vi "Lidar Camera System V2.vi"() -> ()   [LabVIEW 2017]
doc: "This example project provides a library of VIs that work together to wrap various ethernet packet sniffing functions available from WinPcap, a Windows packet capture program.\n\nNote: You must install WinPcap before running this example. You can download WinPcap from www.winpcap.org.\n\nThis VI reads ethernet packets. It outputs the raw data for the packet as a hexadecimal string. It also parses out the ethernet and IP header information, as well as timestamp information for each packet.\n\nThis VI also enumerates all the ethernet adapters on your system and allows you interactively to select between the various adapters.\n\nPlease note that this project is for demonstration purposes only. It was designed to demonstrate one method in which LabVIEW can be used to interface with external software utilities (such as WinPcap). NI Engineers can only address questions on how to call external code from LabVIEW, not the contents of each call demonstrated in this example. In addition, we cannot guarantee that the software will work with newer versions of the external software package."
uses:
  lvwpcap.lvlib
panel:
  out "Filtered Co-ordinates":T1(array[cluster])
  out "3D LIDAR Data":refnum<vi>(3d-picture)
  out "Colour Map":dbl[][](graph)
  in  "No. Points Plotted":i32
  in  "Tab Control":T2(tab)
  in  "Adapters":i32(listbox)
  out "raw data":string
  out "timestamp":cluster{"tv_sec":u32, "tv_usec":u32}
  out "packets":i32
  out "Packet Length":i32
  out "Stored Packet":string
  out "Discarded Packet":string
  out "Identifier":string
  out "Data Points":T3(array[cluster])
  out "Filtered Data (First Filter)":T4(array[cluster])
  out "Coordinates":T1(array[cluster])
  out "Stored Data":T1(array[cluster])
  out "size":i32
  out "Reached Size":bool
  in  "stop":bool
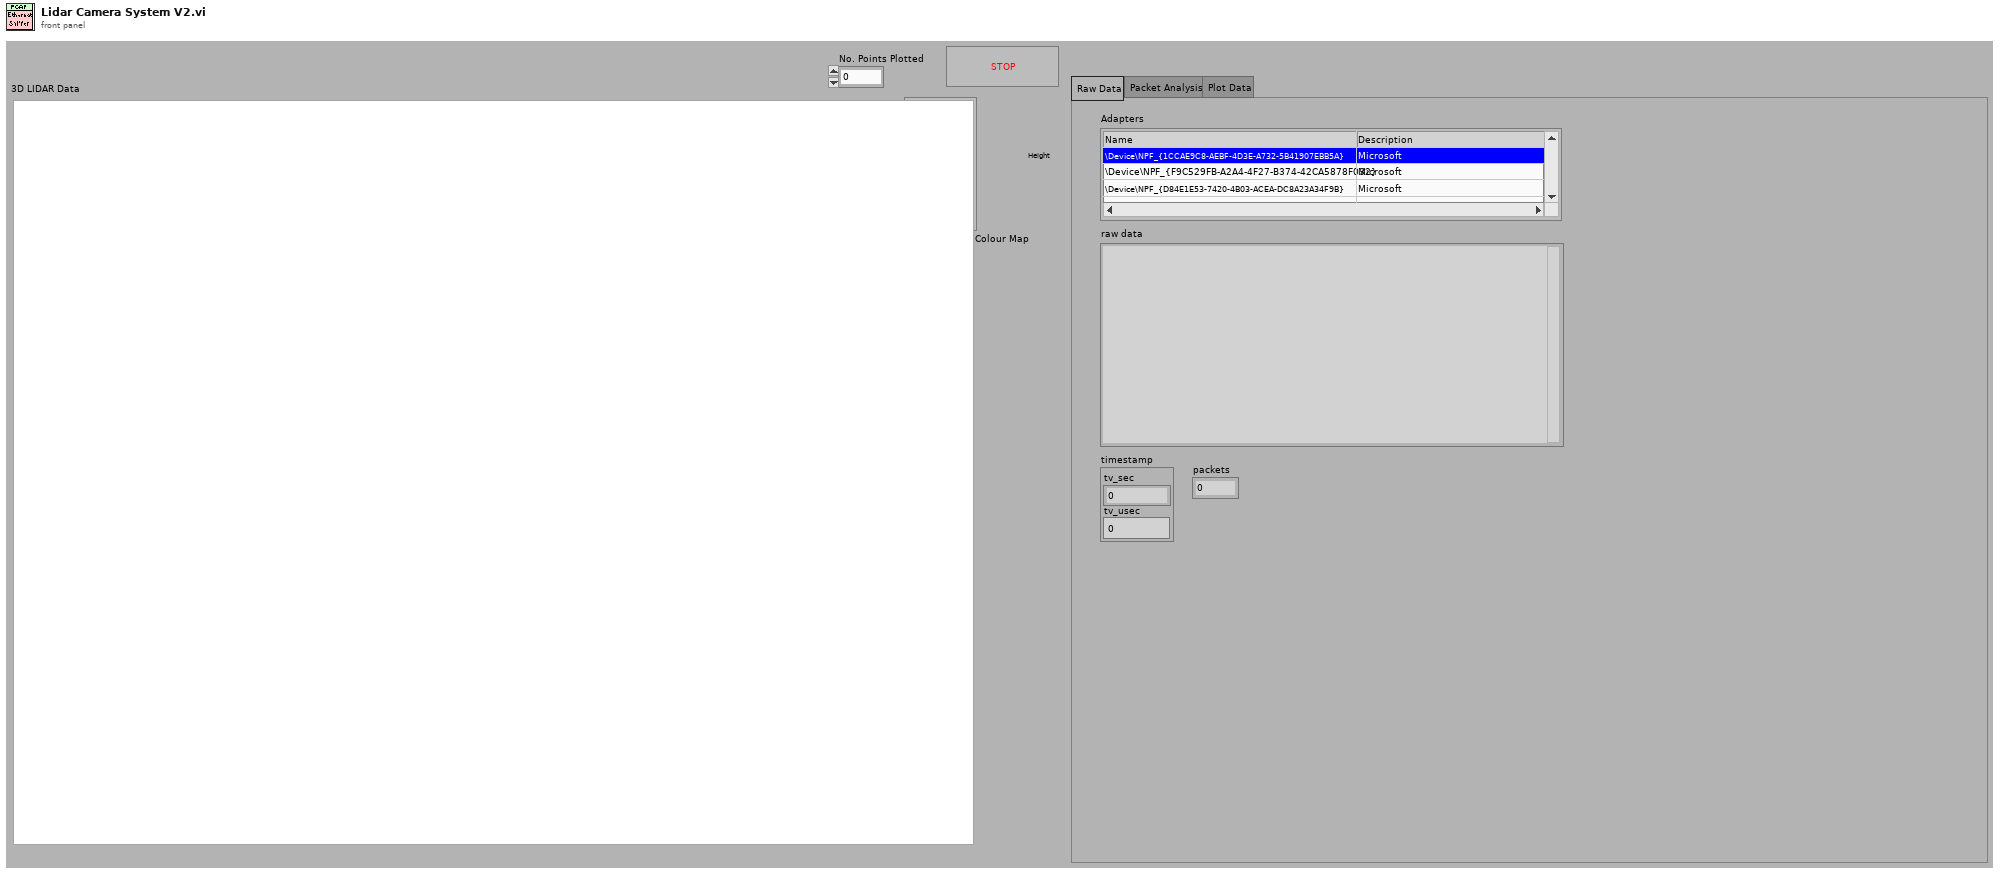
[diagram p1: front panel]
types:
  T1 = cluster{"X":dbl, "Y":dbl, "Z":dbl, "Reflectivity":dbl}[]
  T2 = enum32{"Raw Data", "Packet Analysis", "Plot Data"}
  T3 = cluster{"Azimuth Angle":dbl, "Distance":dbl, "Reflectivity":dbl}[]
  T4 = cluster{"Verticle Angle":dbl, "Azimuth Angle":dbl, "Distance":dbl, "Reflectivity":dbl}[]
  T5 = enum16{"Store Data", "Check Data Size", "Plot Data", "Reinitialise"}
  T6 = enum16{"Check Data", "Check Identifier", "Extract Data", "Filter Data", "Convert to Co-ordinates", "Filter Co-ordinates"}
  T7 = enum16{"Overall", "Per Primitive", "Per Vertex", "Binding Off"}
  T8 = typedef "LVRGBAColorTypeDef.ctl" = cluster{"Red":sgl, "Green":sgl, "Blue":sgl, "Alpha":sgl}
  T9 = enum16{"Check Data", "Check Identifier", "Convert to Hex", "Convert to XYZ", "Check Coords"}
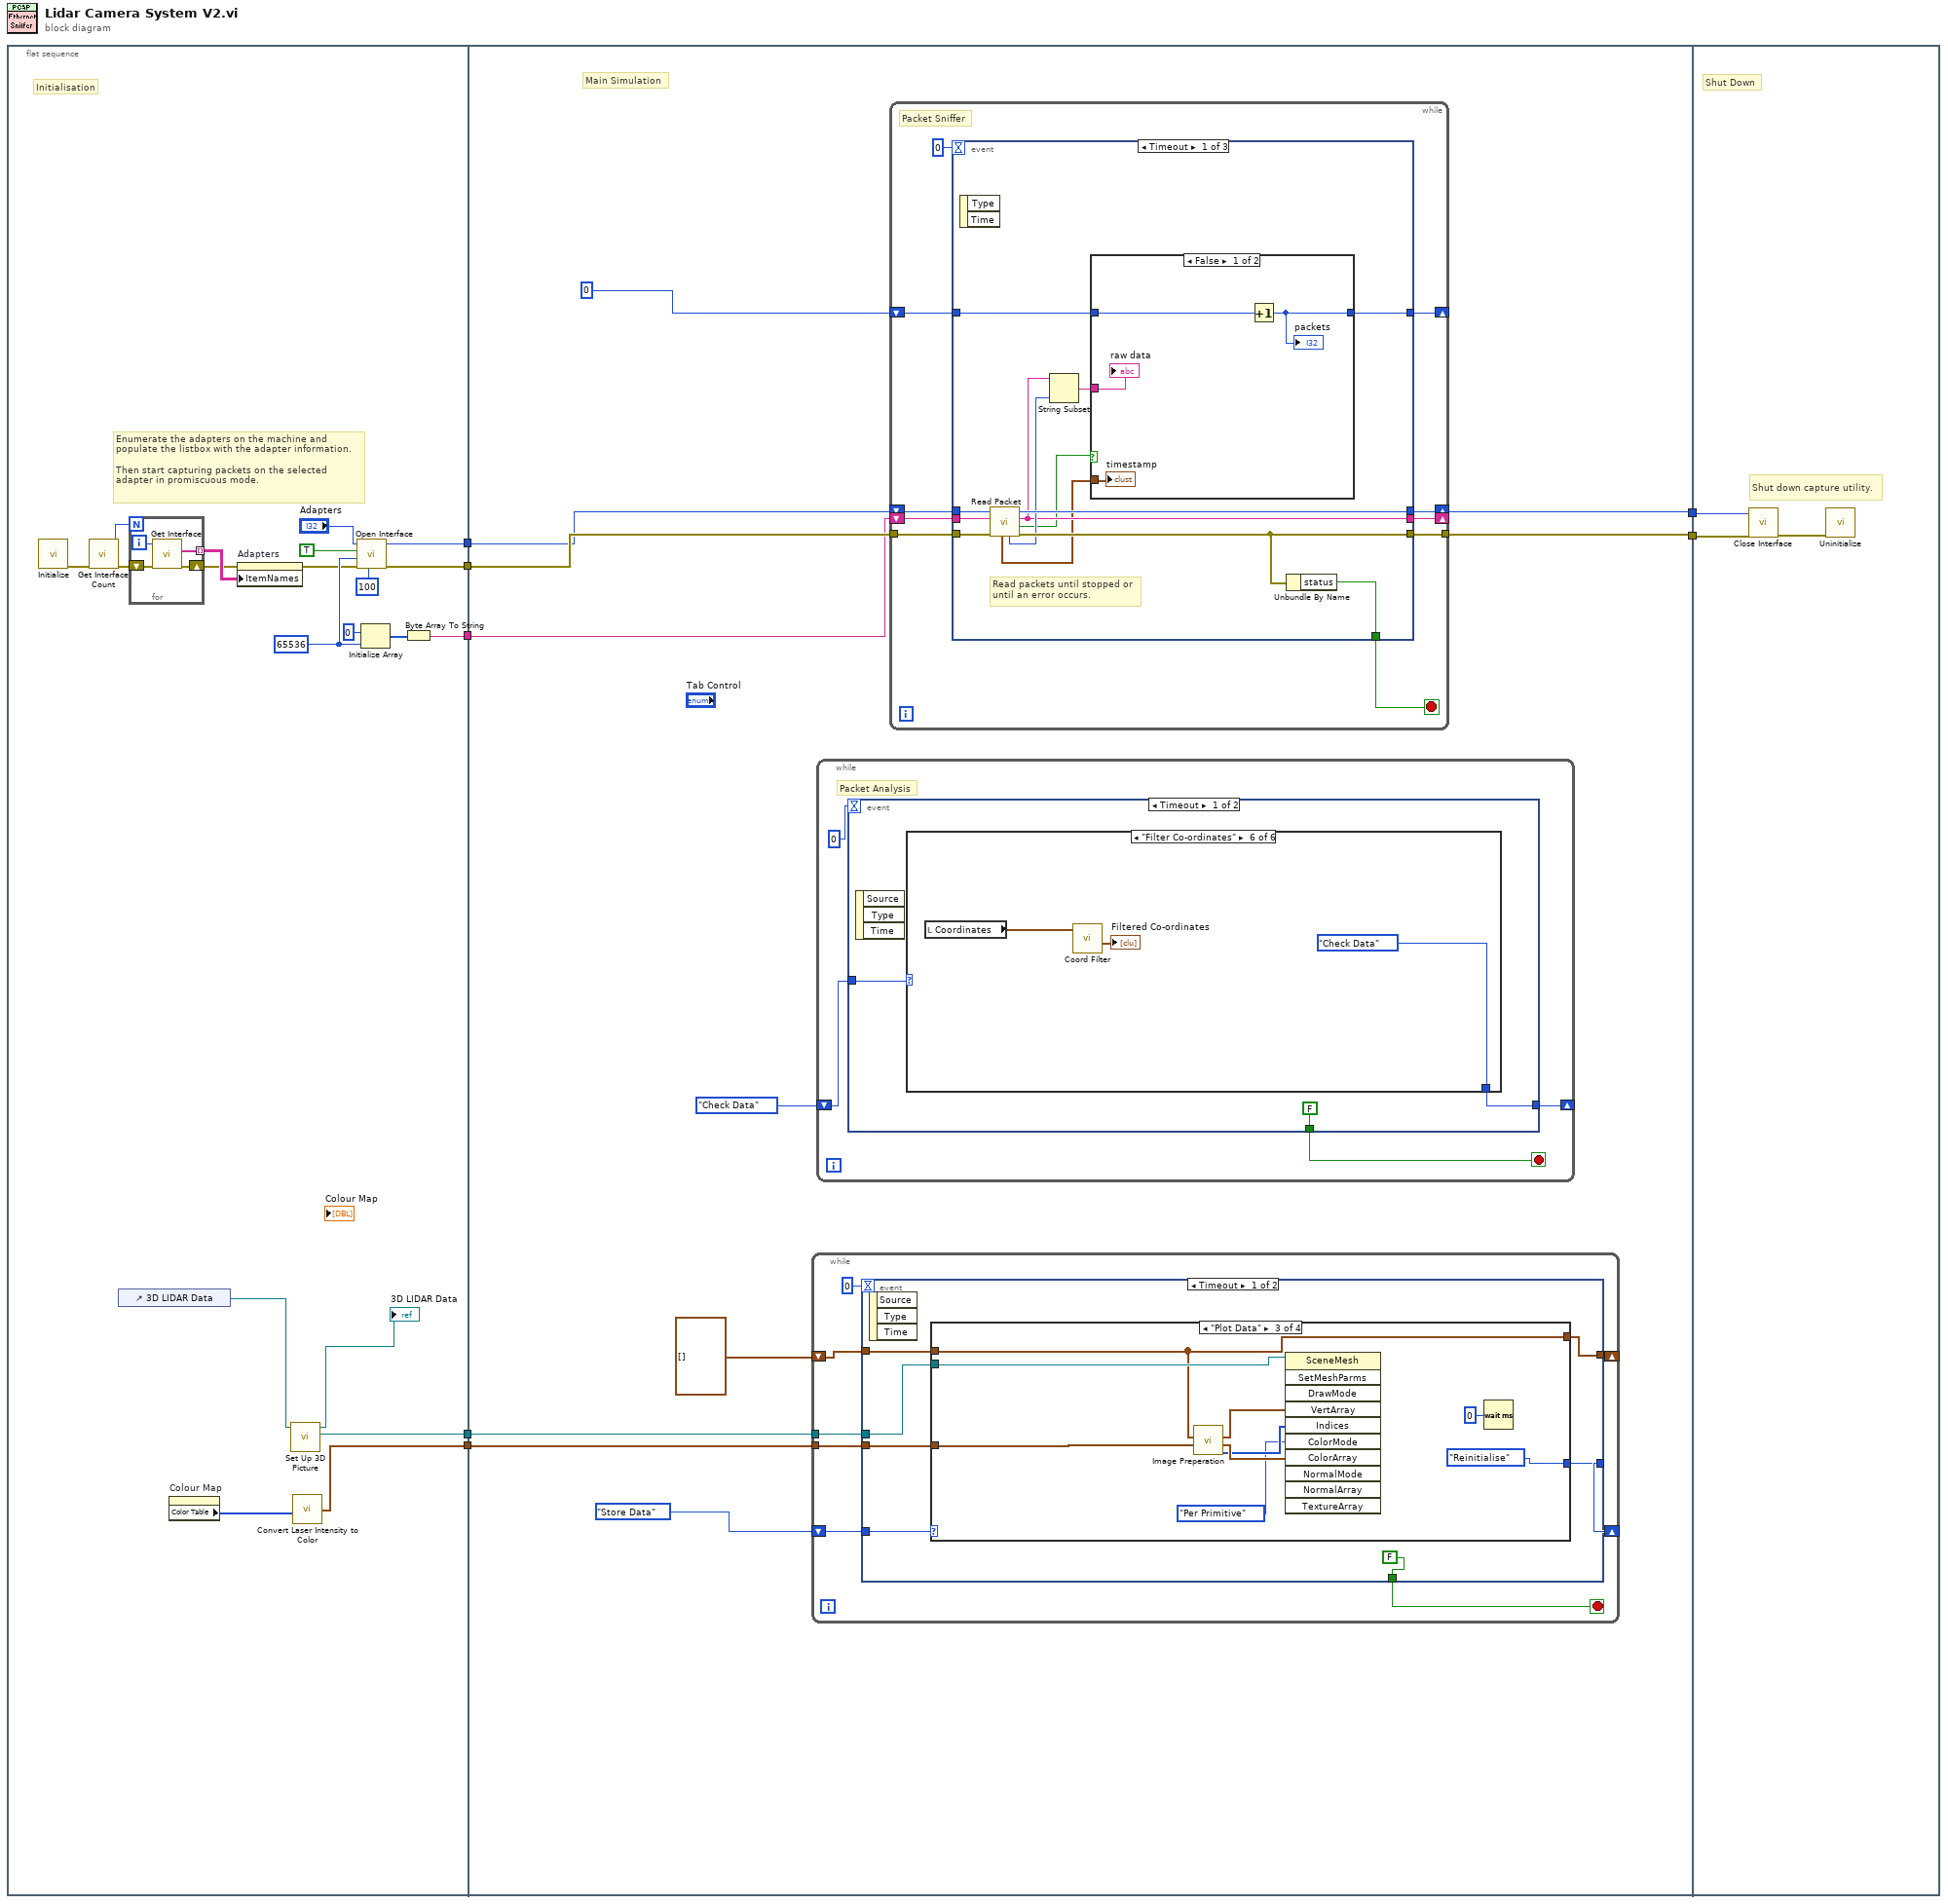
[diagram p0: block diagram]
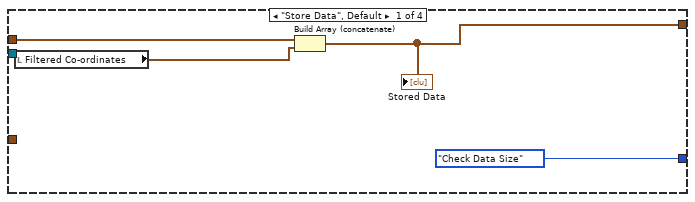
[diagram p2: hidden frame]
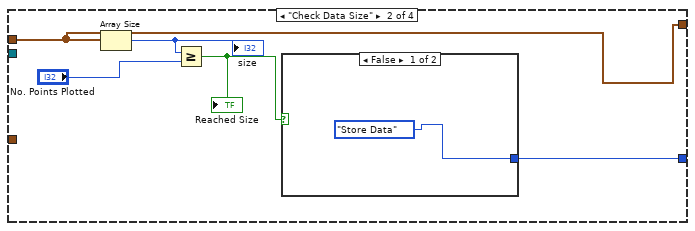
[diagram p3: hidden frame]
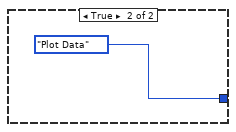
[diagram p4: hidden frame]
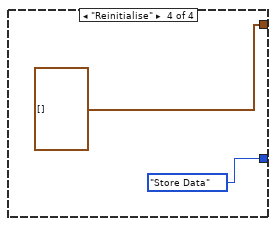
[diagram p5: hidden frame]
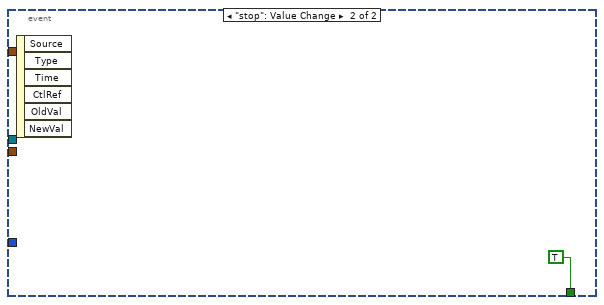
[diagram p6: hidden frame]
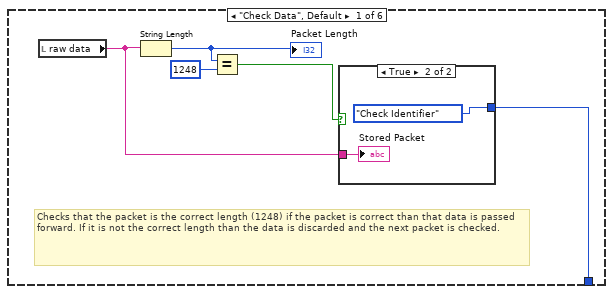
[diagram p7: hidden frame]
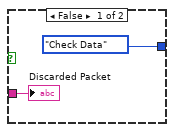
[diagram p8: hidden frame]
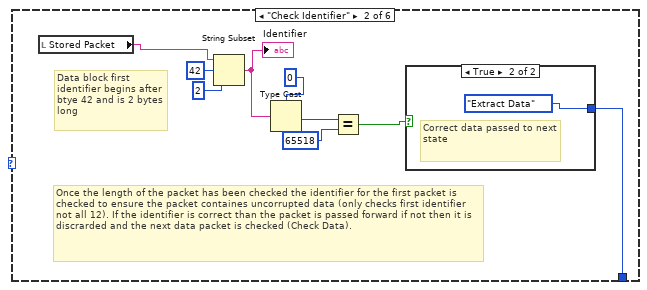
[diagram p9: hidden frame]
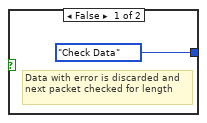
[diagram p10: hidden frame]
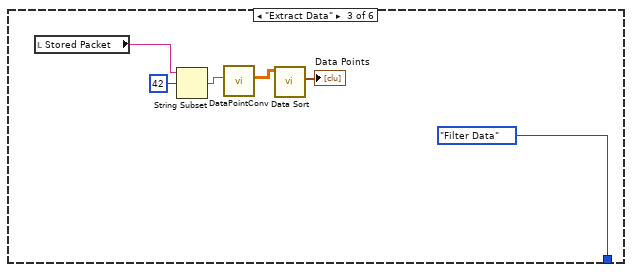
[diagram p11: hidden frame]
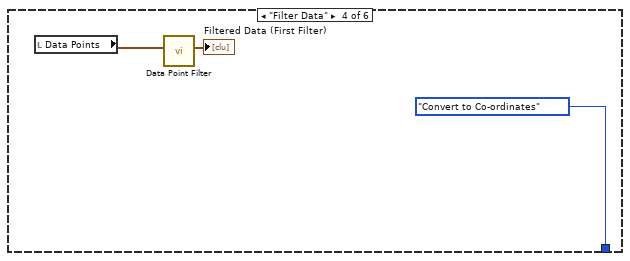
[diagram p12: hidden frame]
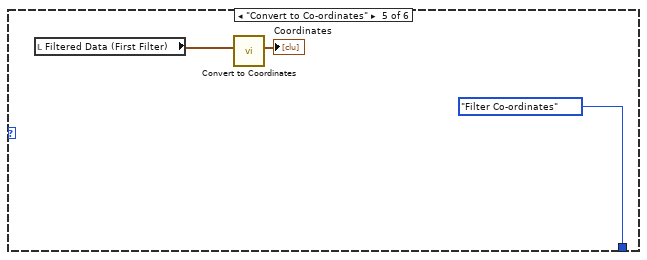
[diagram p13: hidden frame]
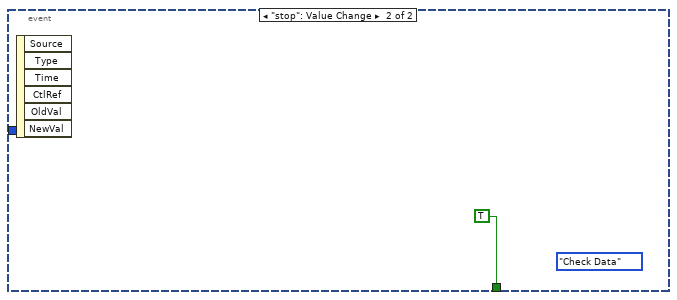
[diagram p14: hidden frame]
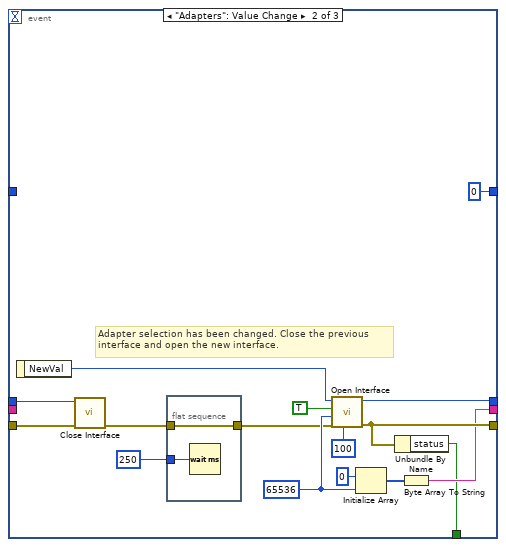
[diagram p16: hidden frame]
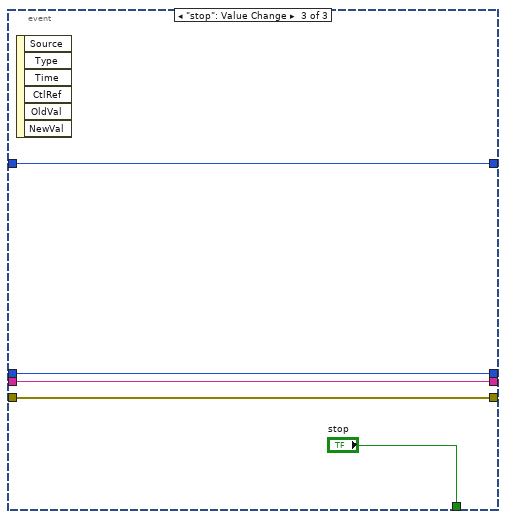
[diagram p17: hidden frame]
diagram:
  n1 = flat-sequence {
    tunnel: [w27] -> w7
    tunnel: [w26] -> w6
    tunnel: [w22] -> w5
    tunnel: [w11] -> w2
    tunnel: [w10] -> w1
    tunnel: w7 -> [w41]
    tunnel: w6 -> [w42]
    tunnel: w5 -> [w40]
    tunnel: [w39] -> w4
    tunnel: [w38] -> w3
    tunnel: w2 -> [w33]
    tunnel: w1 -> [w32]
    tunnel: w4 -> [w177]
    tunnel: w3 -> [w176]
    frame #0 {
      w25 = 65536 ("capture_size (65536)")
      # "Initialisation"
      # "Enumerate the adapters on the machine and\npopulate the listbox with the adapter information.\n\nThen start capturing packets on the selected\nadapter in promiscuous mode."
      n2 = call "Initialize.vi"() -> ("error out"=w20:errorcluster)  [unwired: 11 in]
      n3 = call "Get Interface Count.vi"("error in (no error)"=w20) -> ("error out"=w19:errorcluster, "count"=w18:i32)  [unwired: 9 in]
      n4 = control-ref of="3D LIDAR Data"() -> (w9:refnum<vi>)
      n5 = for {
        N: w18 -> [_]
        shift-right: [w30] -> w14
        shift-left: w19 -> [w31]
        tunnel: [w28] -> w16 mode=indexing
        i -> [w29]
        n6 = call "Get Interface.vi"("error in (no error)"=w31, "index"=w29) -> ("error out"=w30:errorcluster, "lvwpcap_interface_array"=w28:string[])  [unwired: 8 in]
      }
      n7 = property on="Colour Map" class="IntGraph (strict)"() -> ("Color Table"=w12:u32[])  [unwired: 2 in, 2 out]
      n8 = property on="Adapters" class="MCListbox (strict)"(error in=w14, "ItemNames"=w16) -> (error out=w13:errorcluster)  [unwired: 1 in, 1 out]
      n9 = call <instrlib>:"Set Up 3D Picture.vi"("3D Picture Control In"=w9) -> ("Mesh Out"=w11:refnum<vi>, "Scene Out"=→"3D LIDAR Data":refnum<vi>)  [unwired: 9 in]
      n10 = call <instrlib>:"Convert Laser Intensity to Color.vi"("Color Table"=w12) -> ("Color Array"=w10:T8[])  [unwired: 8 in]
      n11 = call "Open Interface.vi"("read_timeout (1000)"=100, "error in (no error)"=w13, "capture_size (65536)"=w25, "promiscuous mode (T)"=TRUE, "adapter (0)"="Adapters") -> ("error out"=w26:errorcluster, "pcap reference"=w27:u32)  [unwired: 5 in]
      n12 = Initialize Array(u8 0, w25) -> (w23:u8[])
      n13 = Byte Array To String(unsigned byte array=w23) -> (string=w22:string)
    }
    frame #1 {
      # "Main Simulation"
      n14 = while {
        shift-right: [w45] -> _
        shift-left: T5."Store Data" -> [w48]
        shift-right: [w46] -> _
        shift-left: cluster{dbl, dbl, dbl, dbl}[] [] -> [w47]
        tunnel: w33 -> [w44]
        tunnel: w32 -> [w43]
        stop <- w49 stop-if-true
        n15 = event shown="[0] Timeout" {
          selector: _ -> [_ _]
          dyn-events: _ -> [_ _]
          timeout: 0 -> [_ _]
          tunnel: [FALSE TRUE] -> w49
          tunnel: w48 -> [w56 _]
          tunnel: w47 -> [w55 _]
          tunnel: [w54 _] -> w46
          tunnel: [w53 _] -> w45
          tunnel: w44 -> [w52 _]
          tunnel: w43 -> [w51 _]
          event Timeout {
            n16 = event-data() -> ()  [unwired: 1 in, 3 out]
            n17 = case shown="\"Plot Data\"" w56 {
              tunnel: w55 -> [w61 w62 w72 _]
              tunnel: [w59 w62 w72 cluster{dbl, dbl, dbl, dbl}[] []] -> w54
              tunnel: [T5."Check Data Size" w63 T5."Reinitialise" T5."Store Data"] -> w53
              tunnel: w52 -> [_ _ w77 _]
              tunnel: w51 -> [_ _ w76 _]
              frame "Store Data", Default {
                n18 = local read "Filtered Co-ordinates"() -> (w60:T1)
                n19 = Build Array (concatenate)(w61, w60) -> (w59:T1)
                "Stored Data" <- w59
              }
              frame "Check Data Size" {
                n20 = Array Size(array=w62) -> (size(s)=w66:i32)
                "size" <- w66
                n21 = Greater Or Equal?(x=w66, y="No. Points Plotted") -> (x >= y?=w64:bool)
                "Reached Size" <- w64
                n22 = case shown="False" w64 {
                  tunnel: [T5."Store Data" T5."Plot Data"] -> w63
                  frame False {
                  }
                  frame True {
                  }
                }
              }
              frame "Plot Data" {
                n23 = call "Image Preperation.vi"("Color Array"=w76, "Coordinates"=w72) -> ("Indicies"=w74:u32[], "Colour"=w75:T8[], "XYZ"=w69:cluster{"X":dbl, "Y":dbl, "Z":dbl}[])  [unwired: 7 in]
                n24 = invoke class="SceneMesh" method="SetMeshParms"(reference=w77, "VertArray"=w69, "Indices"=w74, "ColorMode"=T7."Per Primitive" ("Color Binding Mode"), "ColorArray"=w75) -> ()  [unwired: 6 in, 11 out]
                n25 = Wait (ms)(milliseconds to wait=u32 0) -> ()  [unwired: 1 out]
              }
              frame "Reinitialise" {
              }
            }
          }
          event "stop": Value Change {
            n26 = event-data() -> ()  [unwired: 1 in, 6 out]
          }
        }
      }
      n27 = while {
        shift-right: [w81] -> _
        shift-left: T6."Check Data" -> [w82]
        stop <- w84 stop-if-true
        # "Packet Analysis"
        n28 = event shown="[0] Timeout" {
          selector: _ -> [_ _]
          dyn-events: _ -> [_ _]
          timeout: 0 -> [_ _]
          tunnel: [FALSE TRUE] -> w84
          tunnel: w82 -> [w86 _]
          tunnel: [w85 _] -> w81
          event Timeout {
            n29 = event-data() -> ()  [unwired: 1 in, 3 out]
            n30 = case shown="\"Filter Co-ordinates\"" w86 {
              tunnel: [w88 w97 T6."Filter Data" T6."Convert to Co-ordinates" T6."Filter Co-ordinates" T6."Check Data"] -> w85
              frame "Check Data", Default {
                # "Checks that the packet is the correct length (1248) if the packet is correct than that data is passed forward. If it is not the correct length than the data is discarded and the next packet is checked."
                n31 = local read "raw data"() -> (w89:string)
                n32 = String Length(string=w89) -> (length=w92:i32)
                "Packet Length" <- w92
                n33 = Equal?(x=w92, y=1248) -> (x = y?=w90:bool)
                n34 = case shown="True" w90 {
                  tunnel: w89 -> [w94 w96]
                  tunnel: [T6."Check Data" T6."Check Identifier"] -> w88
                  frame False {
                    "Discarded Packet" <- w94
                  }
                  frame True {
                    "Stored Packet" <- w96
                  }
                }
              }
              frame "Check Identifier" {
                # "Data block first identifier begins after btye 42 and is 2 bytes long"
                # "Once the length of the packet has been checked the identifier for the first packet is checked to ensure the packet containes uncorrupted data (only checks first identifier not all 12). If the identifier is correct than the packet is passed forward if not then it is discrarded and the next data packet is checked (Check Data)."
                n35 = local read "Stored Packet"() -> (w98:string)
                n36 = String Subset(string=w98, offset (0)=42, length (rest)=2 ("length (rest)")) -> (substring=w102:string)
                "Identifier" <- w102
                n37 = Type Cast(type=u16 0, x=w102) -> (*(type *) &x=w100:u16)
                n38 = Equal?(x=w100, y=u16 65518) -> (x = y?=w103:bool)
                n39 = case shown="True" w103 {
                  tunnel: [T6."Check Data" T6."Extract Data"] -> w97
                  frame False {
                    # "Data with error is discarded and next packet checked for length"
                  }
                  frame True {
                    # "Correct data passed to next state"
                  }
                }
              }
              frame "Extract Data" {
                n40 = local read "Stored Packet"() -> (w113:string)
                n41 = String Subset(string=w113, offset (0)=42) -> (substring=w111:string)  [unwired: 1 in]
                n42 = call "DataPointConv.vi"("Stored Data"=w111) -> ("Data Points"=w109:dbl[][])  [unwired: 10 in]
                n43 = call "Data Sort.vi"("Data Points (12 x65)(11x64)"=w109) -> ("Data Points"=→"Data Points":T3)  [unwired: 10 in]
              }
              frame "Filter Data" {
                n44 = local read "Data Points"() -> (w115:T3)
                n45 = call "Data Point Filter.vi"("Data Points"=w115) -> ("Filtered Data"=→"Filtered Data (First Filter)":T4)  [unwired: 10 in]
              }
              frame "Convert to Co-ordinates" {
                n46 = local read "Filtered Data (First Filter)"() -> (w118:T4)
                n47 = call "Convert to Coordinates.vi"("Filtered Data (First Filter)"=w118) -> ("Coordinates"=→"Coordinates":T1)  [unwired: 10 in]
              }
              frame "Filter Co-ordinates" {
                n48 = local read "Coordinates"() -> (w121:T1)
                n49 = call "Coord Filter.vi"("Coordinates"=w121) -> ("Filtered Co-ordinates"=→"Filtered Co-ordinates":T1)  [unwired: 10 in]
              }
            }
          }
          event "stop": Value Change {
            (unwired) T9."Check Data"
            n50 = event-data() -> ()  [unwired: 1 in, 6 out]
          }
        }
      }
      n51 = while {
        tunnel: w42 -> [w132]
        tunnel: [w131] -> w39
        shift-right: [w130] -> w38
        shift-left: w41 -> [w133]
        shift-right: [w128] -> _
        shift-left: w40 -> [w129]
        shift-right: [w126] -> _
        shift-left: 0 -> [w127]
        stop <- w124 stop-if-true
        # "Packet Sniffer"
        n52 = event shown="[0] Timeout" {
          selector: _ -> [_ _ _]
          dyn-events: _ -> [_ _ _]
          timeout: 0 -> [_ _ _]
          tunnel: w133 -> [w146 w154 w173]
          tunnel: w132 -> [w145 w166 w171]
          tunnel: [w144 w167 w171] -> w131
          tunnel: [w143 w164 w173] -> w130
          tunnel: w129 -> [w142 _ w172]
          tunnel: [w140 w159 w172] -> w128
          tunnel: w127 -> [w137 _ w170]
          tunnel: [w136 0 w170] -> w126
          tunnel: [w135 w157 "stop"] -> w124
          event Timeout {
            # "Read packets until stopped or\nuntil an error occurs."
            n53 = event-data() -> ()  [unwired: 1 in, 2 out]
            n54 = call "Read Packet.vi"("error in (no error)"=w145, "capture_data"=w142, "pcap reference"=w146) -> ("error out"=w144:errorcluster, "timed out"=w138:bool, "capture_data out"=w140:string, "pcap reference out"=w143:u32, "capture_len"=w141:u32, "timestamp"=w134:cluster{"tv_sec":u32, "tv_usec":u32})  [unwired: 3 in]
            n55 = String Subset(string=w140, length (rest)=w141) -> (substring=w139:string)  [unwired: 1 in]
            n56 = case shown="False" w138 {
              tunnel: w139 -> [w150 _]
              tunnel: w134 -> [w149 _]
              tunnel: w137 -> [w148 w151]
              tunnel: [w147 w151] -> w136
              frame False {
                n57 = Increment(x=w148) -> (x+1=w147:i32)
                "packets" <- w147
                "raw data" <- w150
                "timestamp" <- w149
              }
              frame True {
                # "timed out"
              }
            }
            n58 = Unbundle By Name(w144) -> ("status"=w135:bool)
          }
          event "Adapters": Value Change {
            w160 = 65536 ("capture_size (65536)")
            # "Adapter selection has been changed. Close the previous\ninterface and open the new interface."
            n59 = event-data() -> ("NewVal"=w165:i32)  [unwired: 1 in]
            n60 = call "Close Interface.vi"("error in (no error)"=w166, "pcap reference"=w154) -> ("error out"=w153:errorcluster)  [unwired: 9 in]
            n61 = flat-sequence {
              tunnel: w153 -> [w169]
              tunnel: [w169] -> w152
              tunnel: u32 250 ("milliseconds to wait") -> [w168]
              frame #0 {
                n62 = Wait (ms)(milliseconds to wait=w168) -> ()  [unwired: 1 out]
              }
            }
            n63 = call "Open Interface.vi"("read_timeout (1000)"=100, "error in (no error)"=w152, "capture_size (65536)"=w160, "promiscuous mode (T)"=TRUE, "adapter (0)"=w165) -> ("error out"=w167:errorcluster, "pcap reference"=w164:u32)  [unwired: 5 in]
            n64 = Initialize Array(u8 0, w160) -> (w162:u8[])
            n65 = Unbundle By Name(w167) -> ("status"=w157:bool)
            n66 = Byte Array To String(unsigned byte array=w162) -> (string=w159:string)
          }
          event "stop": Value Change {
            n67 = event-data() -> ()  [unwired: 1 in, 6 out]
          }
        }
      }
    }
    frame #2 {
      # "Shut Down"
      # "Shut down capture utility."
      n68 = call "Close Interface.vi"("error in (no error)"=w177, "pcap reference"=w176) -> ("error out"=w175:errorcluster)  [unwired: 9 in]
      n69 = call "Uninitialize.vi"("error in (no error)"=w175) -> ()  [unwired: 10 in, 1 out]
    }
  }
